vi "Output single digital pulse.vi"() -> ()   [LabVIEW 2020]
uses:
  <vilib>/Utility/error.llb/DialogType.ctl
  <vilib>/DAQmx/create/channels.llb/DAQmx Create Channel (CO-Pulse Generation-Time).vi
  <resource>/objmgr/daqmx.rc
panel:
  out "elapsed time":dbl
  in  "Pulse Duration":dbl=0.25 format="%.6f"
  in  "Output Terminal":tag="/Dev2/PFI0"
  in  "Counter":tag="Dev2/ctr0"
  in  "Stop":bool
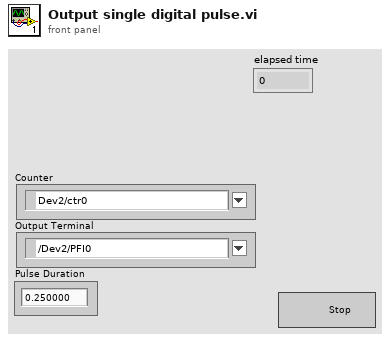
[diagram p1: front panel]
types:
  T1 = typedef "DialogType.ctl" = u16
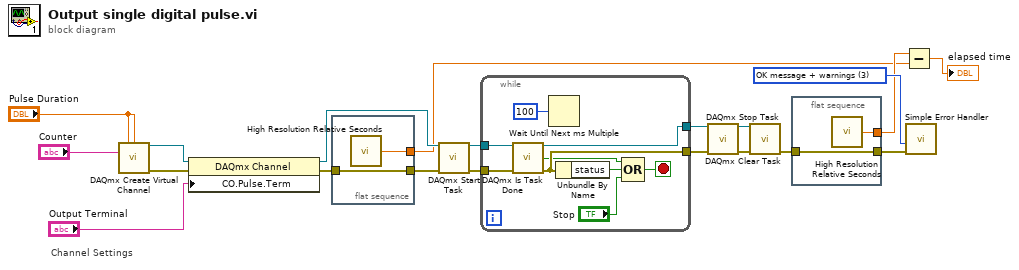
[diagram p0: block diagram]
diagram:
  w8 = T1 3 items=["no dialog", "OK message", "continue or stop message", "OK message + warnings", "continue/stop + warnings"] ("type of dialog (OK msg:1)")
  # "Channel Settings"
  n1 = call-poly <vilib>:"DAQmx Create Virtual Channel.vi"("high time"="Pulse Duration", "low time"="Pulse Duration", "counter"="Counter") -> ("task out"=w17:refnum<k21>, "error out"=w16:errorcluster)  [unwired: 11 in]
  n2 = property class="DAQmx Channel"(reference=w17, error in=w16, "CO.Pulse.Term"="Output Terminal") -> (reference out=w14:refnum<k21>, error out=w7:errorcluster)
  n3 = flat-sequence {
    tunnel: w7 -> [w22]
    tunnel: [w22] -> w6
    tunnel: [w21] -> w2
    frame #0 {
      n4 = call <vilib>:"High Resolution Relative Seconds.vi"() -> ("relative seconds"=w21:dbl)
    }
  }
  n5 = call <vilib>:"DAQmx Start Task.vi"("task/channels in"=w14, "error in"=w6) -> ("task out"=w20:refnum<k21>, "error out"=w19:errorcluster)  [unwired: 12 in]
  n6 = while {
    tunnel: w20 -> [w31]
    tunnel: w19 -> [w30]
    tunnel: [w27] -> w11
    tunnel: [w28] -> w12
    stop <- w29 stop-if-true
    n7 = call <vilib>:"DAQmx Is Task Done.vi"("task/channels in"=w31, "error in"=w30) -> ("task out"=w28:refnum<k21>, "task done?"=w23:bool, "error out"=w27:errorcluster)  [unwired: 11 in]
    n8 = Wait Until Next ms Multiple(millisecond multiple=u32 100) -> ()  [unwired: 1 out]
    n9 = Unbundle By Name(w27) -> ("status"=w26:bool)
    n10 = Compound Arithmetic op=OR(w23, w26, "Stop") -> (w29:bool)
  }
  n11 = call <vilib>:"DAQmx Stop Task.vi"("task/channels in"=w12, "error in"=w11) -> ("task out"=w10:refnum<k21>, "error out"=w9:errorcluster)  [unwired: 12 in]
  n12 = call <vilib>:"DAQmx Clear Task.vi"("task in"=w10, "error in"=w9) -> ("error out"=w5:errorcluster)  [unwired: 13 in]
  n13 = flat-sequence {
    tunnel: w5 -> [w33]
    tunnel: [w33] -> w4
    tunnel: [w32] -> w3
    frame #0 {
      n14 = call <vilib>:"High Resolution Relative Seconds.vi"() -> ("relative seconds"=w32:dbl)
    }
  }
  n15 = Subtract(x=w3, y=w2) -> (x-y=→"elapsed time":dbl)
  n16 = call <vilib>:"Simple Error Handler.vi"("type of dialog (OK msg:1)"=w8, "error in (no error)"=w4) -> ()  [unwired: 3 in, 5 out]
